vi "ColorBox.vi"(10 "Color Box In":u32(colorbox)) -> (2 "Color Box Out":u32)   [LabVIEW 2019]
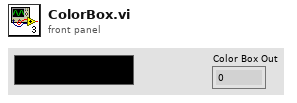
[diagram p1: front panel]
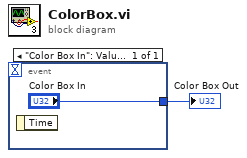
[diagram p0: block diagram]
diagram:
  n1 = event shown="[0] \"Color Box In\": Value Change" {
    selector: _ -> [_]
    dyn-events: _ -> [_]
    timeout: _ -> [_]
    tunnel: ["Color Box In"] -> w1
    event "Color Box In": Value Change {
      n2 = event-data() -> ()  [unwired: 1 in, 1 out]
    }
  }
  "Color Box Out" <- w1
